vi "Connection Validator.vi"(8 "error in (no error)":errorcluster, 10 "VirtualBench Device IO Control":tag) -> (0 "error out":errorcluster, 2 "Passed?":bool)   [LabVIEW 2017]
doc: "Validates the Connections made in the system."
uses:
  <vilib>/VirtualBench/_FGEN Configure Standard Waveform20.vi
  <vilib>/VirtualBench/_PS Configure Voltage Output2.vi
  <vilib>/VirtualBench/_MSO Configure Timing4.vi
  <vilib>/VirtualBench/_MSO Configure Analog Channel30.vi
  <vilib>/measure/matone.llb/Extract Single Tone Information 1 Chan.vi
  <vilib>/VirtualBench/VirtualBench.lvlib
  <vilib>/measure/NI_MAPro.lvlib
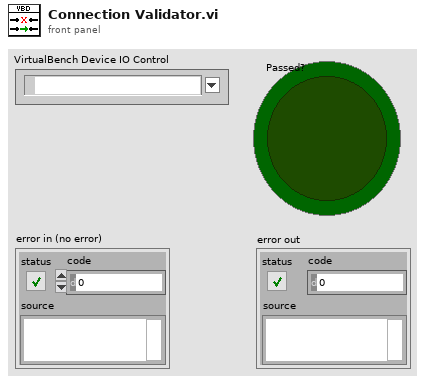
[diagram p1: front panel]
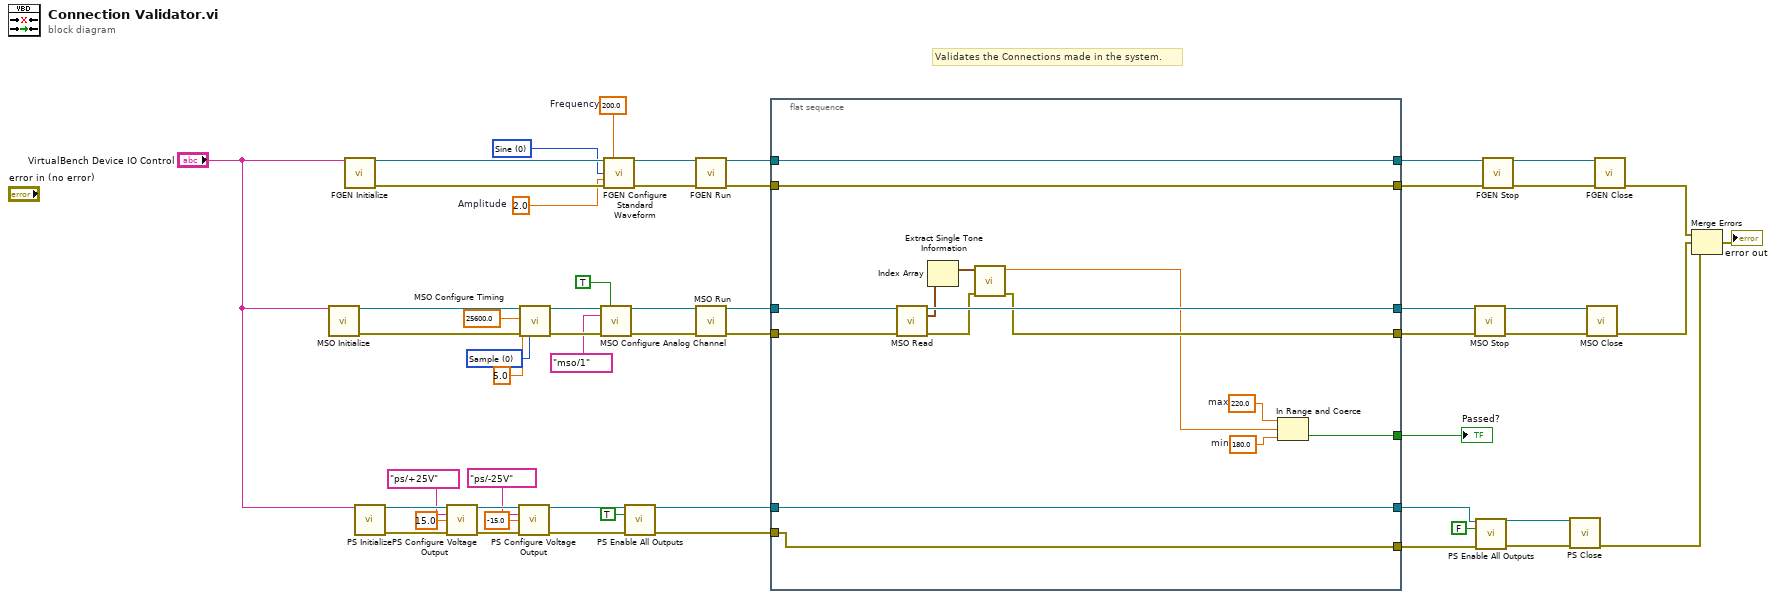
[diagram p0: block diagram]
diagram:
  w37 = 200.0  # Frequency
  w50 = 0 items=["Sine", "Square", "Triangle/Ramp", "DC"] ("Waveform Function")
  w36 = 2.0  # Amplitude
  w38 = 0 items=["Sample", "Peak Detect"] ("Sampling Mode")
  # "Validates the Connections made in the system."
  n1 = call <vilib>:"MSO Initialize.vi"("Device Name"="VirtualBench Device IO Control") -> ("Instrument Handle Out"=w41:refnum<k21>, "Error Out"=w49:errorcluster)  [unwired: 13 in]
  n2 = call <vilib>:"FGEN Initialize.vi"("Device Name"="VirtualBench Device IO Control") -> ("Instrument Handle Out"=w52:refnum<k21>, "Error Out"=w51:errorcluster)  [unwired: 13 in]
  n3 = call <vilib>:"PS Initialize.vi"("Device Name"="VirtualBench Device IO Control") -> ("Instrument Handle Out"=w31:refnum<k21>, "Error Out"=w30:errorcluster)  [unwired: 13 in]
  n4 = call-poly <vilib>:"PS Configure Voltage Output.vi"("Instrument Handle In"=w31, "Channel"=tag "ps/+25V", "Voltage Level"=15.0, "Error In"=w30) -> ("Instrument Handle Out"=w29:refnum<k21>, "Error Out"=w28:errorcluster)  [unwired: 10 in]
  n5 = call-poly <vilib>:"PS Configure Voltage Output.vi"("Instrument Handle In"=w29, "Channel"=tag "ps/-25V", "Voltage Level"=-15.0, "Error In"=w28) -> ("Instrument Handle Out"=w27:refnum<k21>, "Error Out"=w26:errorcluster)  [unwired: 10 in]
  n6 = call-poly <vilib>:"MSO Configure Timing.vi"("Instrument Handle In"=w41, "Sample Rate"=25600.0, "Acquisition Time (s)"=5.0, "Error In"=w49, "Sampling Mode"=w38) -> ("Instrument Handle Out"=w40:refnum<k21>, "Error Out"=w42:errorcluster)  [unwired: 9 in]
  n7 = call-poly <vilib>:"MSO Configure Analog Channel.vi"("Instrument Handle In"=w40, "Enable Channel"=TRUE, "Channel"=tag "mso/1", "Error In"=w42) -> ("Instrument Handle Out"=w12:refnum<k21>, "Error Out"=w13:errorcluster)  [unwired: 10 in]
  n8 = call-poly <vilib>:"FGEN Configure Standard Waveform.vi"("Instrument Handle In"=w52, "Frequency"=w37, "Waveform Function"=w50, "Amplitude"=w36, "Error In"=w51) -> ("Instrument Handle Out"=w11:refnum<k21>, "Error Out"=w10:errorcluster)  [unwired: 9 in]
  n9 = call <vilib>:"PS Enable All Outputs.vi"("Instrument Handle In"=w27, "Enable Outputs"=TRUE, "Error In"=w26) -> ("Instrument Handle Out"=w9:refnum<k21>, "Error Out"=w7:errorcluster)  [unwired: 11 in]
  n10 = call <vilib>:"FGEN Run.vi"("Instrument Handle In"=w11, "Error In"=w10) -> ("Instrument Handle Out"=w5:refnum<k21>, "Error Out"=w3:errorcluster)  [unwired: 12 in]
  n11 = call <vilib>:"MSO Run.vi"("Instrument Handle In"=w12, "Error In"=w13) -> ("Instrument Handle Out"=w48:refnum<k21>, "Error Out"=w47:errorcluster)  [unwired: 12 in]
  n12 = flat-sequence {
    tunnel: w48 -> [w69]
    tunnel: w47 -> [w68]
    tunnel: [w67] -> w46
    tunnel: [w66] -> w45
    tunnel: [w65] -> w35
    tunnel: w9 -> [w58]
    tunnel: [w58] -> w8
    tunnel: w7 -> [w57]
    tunnel: [w57] -> w6
    tunnel: w5 -> [w56]
    tunnel: [w56] -> w4
    tunnel: w3 -> [w55]
    tunnel: [w55] -> w2
    frame #0 {
      w60 = 180.0  # min
      w61 = 220.0  # max
      n13 = call <vilib>:"MSO Read.vi"("Instrument Handle In"=w69, "Error In"=w68) -> ("Instrument Handle Out"=w67:refnum<k21>, "Analog Waveforms"=w63:waveform(dbl)[], "Error Out"=w64:errorcluster)  [unwired: 8 in, 3 out]
      n14 = Index Array(array=w63) -> (element=w62:waveform(dbl))  [unwired: 1 in]
      n15 = call-poly <vilib>:"Extract Single Tone Information.vi"("error in (no error)"=w64, "time signal in"=w62) -> ("error out"=w66:errorcluster, "detected frequency"=w59:dbl)  [unwired: 4 in, 4 out]
      n16 = In Range and Coerce(upper limit=w61, x=w59, lower limit=w60) -> (In Range?=w65:bool)  [unwired: 1 out]
    }
  }
  n17 = call <vilib>:"MSO Stop.vi"("Instrument Handle In"=w46, "Error In"=w45) -> ("Instrument Handle Out"=w44:refnum<k21>, "Error Out"=w43:errorcluster)  [unwired: 12 in]
  n18 = call <vilib>:"PS Enable All Outputs.vi"("Instrument Handle In"=w8, "Enable Outputs"=FALSE, "Error In"=w6) -> ("Instrument Handle Out"=w25:refnum<k21>, "Error Out"=w24:errorcluster)  [unwired: 11 in]
  n19 = call <vilib>:"FGEN Stop.vi"("Instrument Handle In"=w4, "Error In"=w2) -> ("Instrument Handle Out"=w54:refnum<k21>, "Error Out"=w53:errorcluster)  [unwired: 12 in]
  n20 = call <vilib>:"PS Close.vi"("Instrument Handle In"=w25, "Error In"=w24) -> ("Error Out"=w1:errorcluster)  [unwired: 13 in]
  n21 = call <vilib>:"MSO Close.vi"("Instrument Handle In"=w44, "Error In"=w43) -> ("Error Out"=w33:errorcluster)  [unwired: 13 in]
  n22 = call <vilib>:"FGEN Close.vi"("Instrument Handle In"=w54, "Error In"=w53) -> ("Error Out"=w34:errorcluster)  [unwired: 13 in]
  n23 = Merge Errors(w34, w33, w1) -> (→"error out":errorcluster)
  "Passed?" <- w35
